vi "水样测试.vi"(10 "数据标记表":string(combo)="N", 11 "水样测试时间":dbl=1.0) -> ()   [LabVIEW 2016, in "斯坦道多参数.lvlib"]
panel:
  out "运行状态":u16(ring) items=["空闲", "水样测试", "标样核查"]
  out "多参数运行日志":string
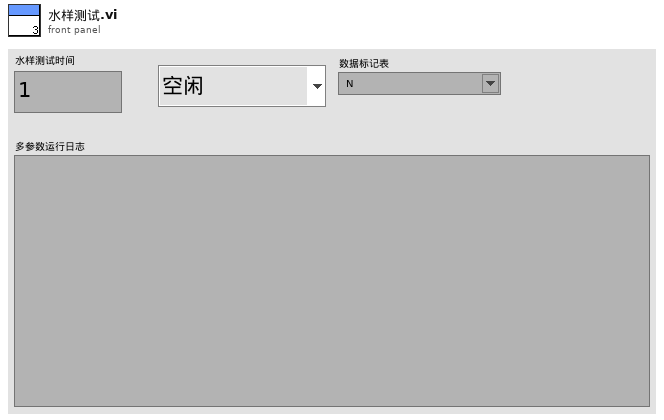
[diagram p1: front panel]
types:
  T1 = cluster{"因子编码":string, "单位":string, "标样参考值":sgl, "水样数据时间":timestamp, "水样实测值":sgl, "水样数据标识":string, "探头温度":sgl}
  T2 = cluster{"CH":u16, "监测值":dbl, "监测信号值":dbl, "温度偏移修正值":sgl}
  T3 = cluster{"电极状态标志":u16, "电极型号标志":u16, "酸碱度测量值":sgl, "温度测量值":sgl, "酸碱度信号值":sgl, "温度信号值":sgl, "酸碱度偏移修正值":sgl, "温度偏移修正值":sgl, "手动温度补偿值":sgl, "酸碱度电极零点":sgl, "酸碱度电极斜率":sgl, "第1点标准值记录":sgl, "第1点信号值记录":sgl, "第1点温度值记录":sgl, "第2点标准值记录":sgl, "第2点信号值记录":sgl, "第2点温度值记录":sgl, "命令滤波设定":u16, "温度模式":enum16{"ATC", "MTC"}, "生产批次":u16, "电极序号":u16, "串口地址":u16, "串口波特率":enum16{"9600", "19200", "115200"}, "串口校验位":enum16{"NONE", "ODD", "EVEN"}, "串口停止位":enum16{"1bit", "2bit"}, "第一点标准值":sgl, "第二点标准值":sgl}
  T4 = cluster{"电极状态标志":u16, "电极型号标志":u16, "溶解氧测量值":sgl, "温度测量值":sgl, "溶解氧饱和度值":sgl, "盐度补偿值":sgl, "大气压补偿值":sgl, "溶解氧偏移修正值":sgl, "温度偏移修正值":sgl, "手动温度补偿值":sgl, "溶解氧电极零点":sgl, "溶解氧电极斜率":sgl, "第1点标准值记录":sgl, "第1点信号值记录":sgl, "第1点温度值记录":sgl, "第2点标准值记录":sgl, "第2点信号值记录":sgl, "第2点温度值记录":sgl, "命令滤波设定":u16, "温度模式":enum16{"ATC", "MTC"}, "生产批次":u16, "电极序号":u16, "串口地址":u16, "串口波特率":enum16{"9600", "19200", "115200"}, "串口校验位":enum16{"NONE", "ODD", "EVEN"}, "串口停止位":enum16{"1bit", "2bit"}, "第一点标准值":sgl, "第二点标准值":sgl}
  T5 = cluster{"电极状态标志":u16, "电极型号标志":u16, "电导率测量值":sgl, "温度测量值":sgl, "电导率信号值":sgl, "温度信号值":sgl, "温度补偿系数":sgl, "电导率偏移修正值":sgl, "温度偏移修正值":sgl, "手动温度补偿值":sgl, "电导率电极零点":sgl, "电导率电极斜率":sgl, "命令滤波设定":u16, "温度模式":enum16{"ATC", "MTC"}, "生产批次":u16, "电极序号":u16, "串口地址":u16, "串口波特率":enum16{"9600", "19200", "115200"}, "串口校验位":enum16{"NONE", "ODD", "EVEN"}, "串口停止位":enum16{"1bit", "2bit"}, "第一点标准值":sgl, "第二点标准值":sgl}
  T6 = cluster{"电极状态标志":u16, "电极型号标志":u16, "浊度测量值":sgl, "温度测量值":sgl, "浊度信号值":sgl, "浊度偏移修正值":sgl, "温度偏移修正值":sgl, "手动温度补偿值":sgl, "浊度电极零点":sgl, "浊度电极斜率":sgl, "第1点标准值记录":sgl, "第1点信号值记录":sgl, "第1点温度值记录":sgl, "第2点标准值记录":sgl, "第2点信号值记录":sgl, "第2点温度值记录":sgl, "命令滤波设定":u16, "温度模式":enum16{"ATC", "MTC"}, "生产批次":u16, "电极序号":u16, "串口地址":u16, "串口波特率":enum16{"9600", "19200", "115200"}, "串口校验位":enum16{"NONE", "ODD", "EVEN"}, "串口停止位":enum16{"1bit", "2bit"}, "第一点标准值":sgl, "第二点标准值":sgl}
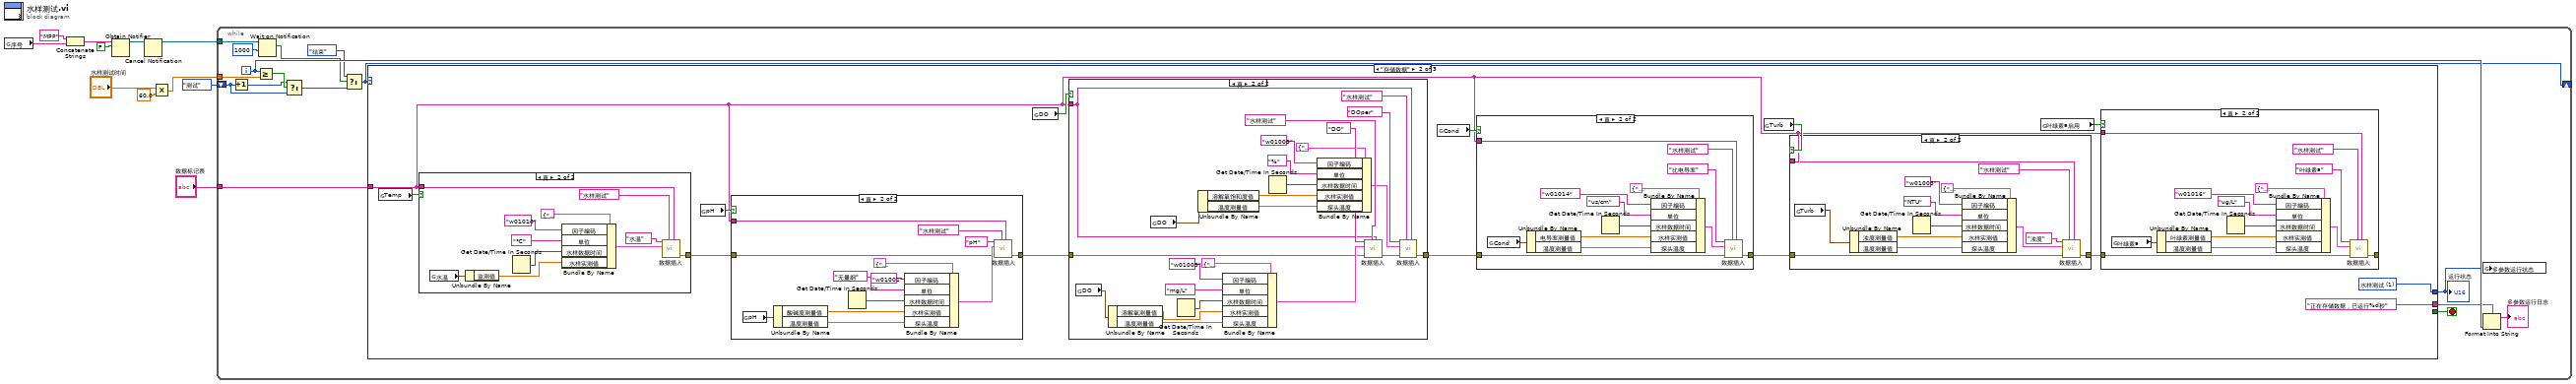
[diagram p0: block diagram]
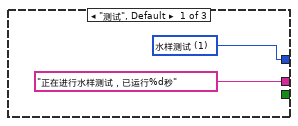
[diagram p2: hidden frame]
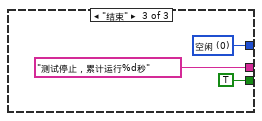
[diagram p9: hidden frame]
diagram:
  n1 = global read "多参数全局变量.vi" "序号"() -> (w1:string)
  n2 = Concatenate Strings("MPP" ("名称（未命名）"), w1) -> (w2:string)
  n3 = Obtain Notifier(name (unnamed)=w2, notification data type=FALSE) -> (notifier out=w5:refnum<notifier>)  [unwired: 2 in, 2 out]
  n4 = Cancel Notification(0:w5) -> (8:w4:refnum<notifier>)  [unwired: 1 in, 2 out]
  n5 = Multiply(x="水样测试时间", y=60.0) -> (x*y=w9:dbl)
  n6 = while {
    tunnel: w9 -> [w27]
    shift-right: [w14] -> _
    shift-left: enum16{"测试", "存储数据", "结束"}."测试" ("枚举") -> [w21]
    tunnel: w4 -> [w19]
    tunnel: "数据标记表" -> [w13]
    i -> [w25]
    stop <- w26 stop-if-true
    n7 = Increment(x=w21) -> (x+1=w20:enum16{"测试", "存储数据", "结束"})
    n8 = Greater Or Equal?(x=w25, y=w27) -> (x >= y?=w22:bool)
    n9 = Wait on Notification(notifier=w19, timeout in ms (-1)=1000 ("超时毫秒(-1)")) -> (notification=w17:bool)  [unwired: 2 in, 3 out]
    n10 = Select(t=w20, s=w22, f=w21) -> (s? t:f=w15:enum16{"测试", "存储数据", "结束"})
    n11 = Select(t=enum16{"测试", "存储数据", "结束"}."结束" ("枚举"), s=w17, f=w15) -> (s? t:f=w14:enum16{"测试", "存储数据", "结束"})
    n12 = case shown="\"存储数据\"" w14 {
      tunnel: [_ _ TRUE] -> w26
      tunnel: ["正在进行水样测试，已运行%d秒" ("格式字符串") "正在存储数据，已运行%d秒" ("格式字符串") "测试停止，累计运行%d秒" ("格式字符串")] -> w24
      tunnel: [w28 w31 w131] -> w12
      tunnel: w13 -> [_ w30 _]
      frame "测试", Default {
        w28 = u16 1 items=["空闲", "水样测试", "标样核查"] ("多参数运行状态")
      }
      frame "存储数据" {
        w31 = u16 1 items=["空闲", "水样测试", "标样核查"] ("多参数运行状态")
        n13 = global read "断电保存变量.vi" "Temp"() -> (w38:bool)
        n14 = case shown="真" w38 {
          tunnel: [_ w121] -> w33
          tunnel: w30 -> [_ w120]
          frame False {
          }
          frame True {
            n15 = global read "国弘过程全局变量.vi" "水温"() -> (w129:T2)
            n16 = Unbundle By Name(w129) -> ("监测值"=w128:dbl)
            n17 = Get Date/Time In Seconds() -> (seconds since 1Jan1904=w127:timestamp)
            n18 = Bundle By Name(cluster=T1 {"因子编码"="w01003", "单位"="无量纲", "标样参考值"=0.0, "水样数据时间"=timestamp(0 s since 1904-01-01), "水样实测值"=0.0, "水样数据标识"="N", "探头温度"=0.0} ("data in"), "因子编码"="w01010", "单位"="℃", "水样数据时间"=w127, "水样实测值"=w128) -> (w126:T1)
            n19 = call "数据插入.vi"("数据标记表"=w120, "测量模式"="水样测试", "data in"=w126, "table输入"="水温") -> ("error out"=w121:errorcluster)  [unwired: 7 in]
          }
        }
        n20 = global read "断电保存变量.vi" "pH"() -> (w39:bool)
        n21 = case shown="真" w39 {
          tunnel: w33 -> [_ w109]
          tunnel: [_ w108] -> w34
          tunnel: w30 -> [_ w107]
          frame False {
          }
          frame True {
            n22 = global read "国弘过程全局变量.vi" "pH"() -> (w115:T3)
            n23 = Unbundle By Name(w115) -> ("酸碱度测量值"=w116:sgl, "温度测量值"=w113:sgl)
            n24 = Get Date/Time In Seconds() -> (seconds since 1Jan1904=w117:timestamp)
            n25 = Bundle By Name(cluster=T1 {"因子编码"="w01003", "单位"="无量纲", "标样参考值"=0.0, "水样数据时间"=timestamp(0 s since 1904-01-01), "水样实测值"=0.0, "水样数据标识"="N", "探头温度"=0.0} ("data in"), "因子编码"="w01001", "单位"="无量纲", "水样数据时间"=w117, "水样实测值"=w116, "探头温度"=w113) -> (w118:T1)
            n26 = call "数据插入.vi"("数据标记表"=w107, "测量模式"="水样测试", "error in (no error)"=w109, "data in"=w118, "table输入"="pH") -> ("error out"=w108:errorcluster)  [unwired: 6 in]
          }
        }
        n27 = global read "断电保存变量.vi" "DO"() -> (w40:bool)
        n28 = case shown="真" w40 {
          tunnel: w34 -> [_ w97]
          tunnel: [_ w95] -> w35
          tunnel: w30 -> [_ w93]
          frame False {
          }
          frame True {
            n29 = global read "国弘过程全局变量.vi" "DO"() -> (w84:T4)
            n30 = Unbundle By Name(w84) -> ("溶解氧测量值"=w104:sgl, "温度测量值"=w106:sgl)
            n31 = global read "国弘过程全局变量.vi" "DO"() -> (w83:T4)
            n32 = Get Date/Time In Seconds() -> (seconds since 1Jan1904=w103:timestamp)
            n33 = Unbundle By Name(w83) -> ("溶解氧饱和度值"=w88:sgl, "温度测量值"=w86:sgl)
            n34 = Bundle By Name(cluster=T1 {"因子编码"="w01003", "单位"="无量纲", "标样参考值"=0.0, "水样数据时间"=timestamp(0 s since 1904-01-01), "水样实测值"=0.0, "水样数据标识"="N", "探头温度"=0.0} ("data in"), "因子编码"="w01009", "单位"="mg/L", "水样数据时间"=w103, "水样实测值"=w104, "探头温度"=w106) -> (w102:T1)
            n35 = Get Date/Time In Seconds() -> (seconds since 1Jan1904=w89:timestamp)
            n36 = Bundle By Name(cluster=T1 {"因子编码"="w01003", "单位"="无量纲", "标样参考值"=0.0, "水样数据时间"=timestamp(0 s since 1904-01-01), "水样实测值"=0.0, "水样数据标识"="N", "探头温度"=0.0} ("data in"), "因子编码"="w01009", "单位"="%", "水样数据时间"=w89, "水样实测值"=w88, "探头温度"=w86) -> (w85:T1)
            n37 = call "数据插入.vi"("数据标记表"=w93, "测量模式"="水样测试", "error in (no error)"=w97, "data in"=w102, "table输入"="DO") -> ("error out"=w96:errorcluster)  [unwired: 6 in]
            n38 = call "数据插入.vi"("数据标记表"=w93, "测量模式"="水样测试", "error in (no error)"=w96, "data in"=w85, "table输入"="DOper") -> ("error out"=w95:errorcluster)  [unwired: 6 in]
          }
        }
        n39 = global read "断电保存变量.vi" "Cond"() -> (w41:bool)
        n40 = case shown="真" w41 {
          tunnel: w35 -> [_ w72]
          tunnel: [_ w71] -> w36
          tunnel: w30 -> [_ w70]
          frame False {
          }
          frame True {
            n41 = global read "国弘过程全局变量.vi" "Cond"() -> (w78:T5)
            n42 = Unbundle By Name(w78) -> ("电导率测量值"=w79:sgl, "温度测量值"=w76:sgl)
            n43 = Get Date/Time In Seconds() -> (seconds since 1Jan1904=w80:timestamp)
            n44 = Bundle By Name(cluster=T1 {"因子编码"="w01003", "单位"="无量纲", "标样参考值"=0.0, "水样数据时间"=timestamp(0 s since 1904-01-01), "水样实测值"=0.0, "水样数据标识"="N", "探头温度"=0.0} ("data in"), "因子编码"="w01014", "单位"="us/cm", "水样数据时间"=w80, "水样实测值"=w79, "探头温度"=w76) -> (w81:T1)
            n45 = call "数据插入.vi"("数据标记表"=w70, "测量模式"="水样测试", "error in (no error)"=w72, "data in"=w81, "table输入"="比电导率") -> ("error out"=w71:errorcluster)  [unwired: 6 in]
          }
        }
        n46 = global read "断电保存变量.vi" "Turb"() -> (w42:bool)
        n47 = case shown="真" w42 {
          tunnel: w36 -> [_ w60]
          tunnel: [_ w59] -> w37
          tunnel: w30 -> [_ w58]
          frame False {
          }
          frame True {
            n48 = global read "国弘过程全局变量.vi" "Turb"() -> (w57:T6)
            n49 = Unbundle By Name(w57) -> ("浊度测量值"=w67:sgl, "温度测量值"=w69:sgl)
            n50 = Get Date/Time In Seconds() -> (seconds since 1Jan1904=w66:timestamp)
            n51 = Bundle By Name(cluster=T1 {"因子编码"="w01003", "单位"="无量纲", "标样参考值"=0.0, "水样数据时间"=timestamp(0 s since 1904-01-01), "水样实测值"=0.0, "水样数据标识"="N", "探头温度"=0.0} ("data in"), "因子编码"="w01003", "单位"="NTU", "水样数据时间"=w66, "水样实测值"=w67, "探头温度"=w69) -> (w65:T1)
            n52 = call "数据插入.vi"("数据标记表"=w58, "测量模式"="水样测试", "error in (no error)"=w60, "data in"=w65, "table输入"="浊度") -> ("error out"=w59:errorcluster)  [unwired: 6 in]
          }
        }
        n53 = global read "断电保存变量.vi" "叶绿素a启用"() -> (w43:bool)
        n54 = case shown="真" w43 {
          tunnel: w37 -> [_ w47]
          tunnel: [_ w46] -> _
          tunnel: w30 -> [_ w45]
          frame False {
          }
          frame True {
            n55 = global read "禹山过程全局变量.vi" "叶绿素a"() -> (w44:cluster{"温度测量值":sgl, "叶绿素测量值":sgl, "错误标志":u16})
            n56 = Unbundle By Name(w44) -> ("叶绿素测量值"=w54:sgl, "温度测量值"=w52:sgl)
            n57 = Get Date/Time In Seconds() -> (seconds since 1Jan1904=w55:timestamp)
            n58 = Bundle By Name(cluster=T1 {"因子编码"="w01003", "单位"="无量纲", "标样参考值"=0.0, "水样数据时间"=timestamp(0 s since 1904-01-01), "水样实测值"=0.0, "水样数据标识"="N", "探头温度"=0.0} ("data in"), "因子编码"="w01016", "单位"="ug/L", "水样数据时间"=w55, "水样实测值"=w54, "探头温度"=w52) -> (w50:T1)
            n59 = call "数据插入.vi"("数据标记表"=w45, "测量模式"="水样测试", "error in (no error)"=w47, "data in"=w50, "table输入"="叶绿素a") -> ("error out"=w46:errorcluster)  [unwired: 6 in]
          }
        }
      }
      frame "结束" {
        w131 = u16 0 items=["空闲", "水样测试", "标样核查"] ("多参数运行状态")
      }
    }
    "运行状态" <- w12
    n60 = global write "多参数全局变量.vi" "多参数运行状态"(w12) -> ()
    n61 = Format Into String(format string=w24, w25) -> (resulting string=→"多参数运行日志":string)  [unwired: 2 in, 1 out]
  }
